vi "FTW-HTTPClient-POST.vi"(0 "HTTP Client":refnum<class "FTW-HTTPClient.lvclass">, 5 "Endpoint":string, 7 "Request Payload":string, 11 "error in":errorcluster) -> (4 "HTTP Client out":refnum<class "FTW-HTTPClient.lvclass">, 6 "Response Headers":string, 8 "Response Body":string, 15 "error out":errorcluster)   [LabVIEW 2015, in "FTW-HTTPClient.lvclass"]
uses:
  FTW-HTTPClient.lvclass
  FTW-HTTPClient.lvclass/FTW-HTTPClient.ctl
  error/FTW-ERR-CallChain.vi
  error/FTW-ERR-NoErrorConstant.vi
  string/FTW-STR-ReplaceWhitespace.vi
  string/FTW-STR-Array-Delimit.vi
  error/FTW-ERR-Clear.vi
  regex/FTW-Regex-ReplaceAll.vi
panel:
  # "Inputs"
  # "Outputs"
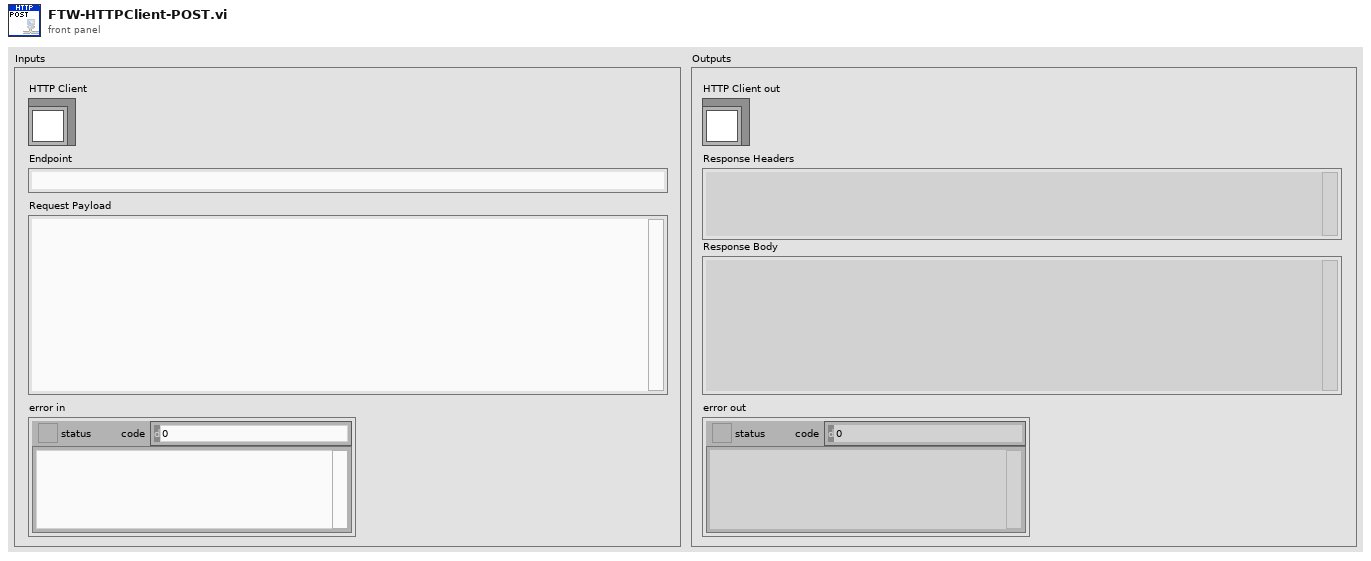
[diagram p1: front panel]
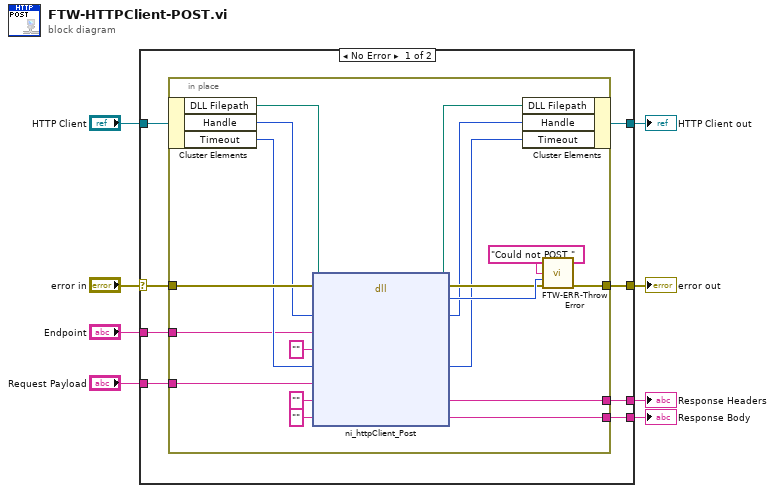
[diagram p0: block diagram]
diagram:
  n1 = case shown="No Error" "error in" {
    selector: "error in" -> [w15 w36]
    tunnel: "Endpoint" -> [w13 _]
    tunnel: [w11 w36] -> w7
    tunnel: "HTTP Client" -> [w16 w35]
    tunnel: [w14 w35] -> w6
    tunnel: "Request Payload" -> [w12 _]
    tunnel: [w10 _] -> w2
    tunnel: [w9 _] -> w1
    frame No Error {
      n2 = in-place {
        in-place-border: w15 -> [w34]
        in-place-border: w13 -> [w26]
        in-place-border: w12 -> [w25]
        in-place-border: [w28] -> w11
        in-place-border: [w22] -> w10
        in-place-border: [w21] -> w9
        n3 = in-place-cluster #1(w16) -> ("DLL Filepath"=w33:path, "Handle"=w19:u32, "Timeout"=w27:i32)
        n4 = dll-call lib="?" fn="ni_httpClient_Post"(path in=w33, error in=w34, "Handle"=w19, "Endpoint"=w26, "Output Filepath"="", "Timeout"=w27, "Request Payload"=w25, "Response Header"="", "Response Body"="") -> (path out=w32:path, error out=w30:errorcluster, "Return"=w31:i32, "Handle"=w18:u32, "Timeout"=w17:i32, "Response Header"=w22:string, "Response Body"=w21:string)  [unwired: 4 in]
        n5 = in-place-cluster #1("DLL Filepath"=w32, "Handle"=w18, "Timeout"=w17) -> (w14:refnum<class "FTW-HTTPClient.lvclass">)
        n6 = call "FTW-ERR-ThrowError.vi"("Error Message"="Could not POST.", "Error Code"=w31, "error in"=w30) -> ("error out"=w28:errorcluster)  [unwired: 12 in]
      }
    }
    frame Error {
    }
  }
  "error out" <- w7
  "HTTP Client out" <- w6
  "Response Headers" <- w2
  "Response Body" <- w1
